vi "ST5 Read Param.vi"(6 "Facteur Dir":bool, 8 "error in (no error)":errorcluster, 9 "Facteur Pas":dbl=1500.0, 10 "Parameters":u16(ring) items=["All", "Velocity", "Acceleration", "Deceleration", "Max Acceleration", "Position", "Step/Rev", "Alarm Code", "Status"], 11 "Port COM":refnum<visa-resource-name>) -> (0 "error out":errorcluster, 1 "Status":T1, 2 "Position":dbl caption="Position (mm)" min=0.0 max=119304.64 step=0.018 format="%#.4g", 3 "Port COM Out":refnum<visa-resource-name>, 4 "Speed Par":T2 {"Accél Max" min=0.167 max=5461.167 step=0.167 format="%#.3g"; "Décél" min=0.167 max=5461.167 step=0.167 format="%#.3g"; "Accél" min=0.167 max=5461.167 step=0.167 format="%#.3g"; "Vitesse (Tour/s)" min=0.0042 max=133.3333 step=0.0042 format="%#.4g"}, 5 "Résolution Pas":dbl, 7 "Alarme":u32)   [LabVIEW 2010]
doc: "Ce Vi envoie les chaînes de commande au contrôlleur de moteur ST5-Q et vérifie si une réponse se trouve dans le buffer du port série"
uses:
  <userlib>/ST5/StatesConst.ctl
panel:
  out "ScanFailed":bool
  out "Réponse":string
  out "Commande":string
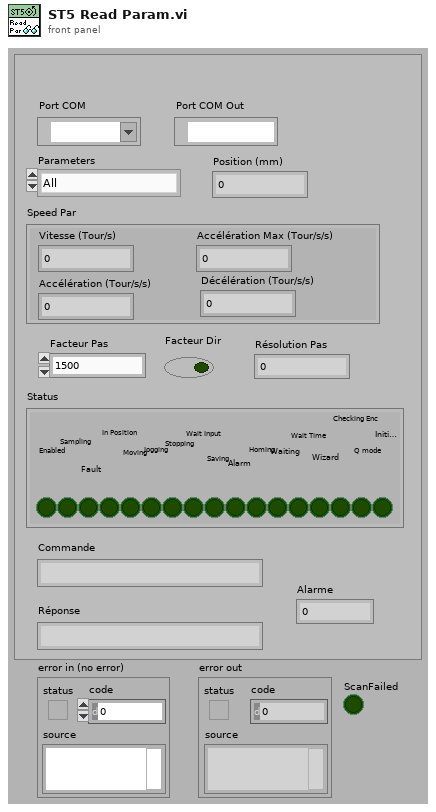
[diagram p1: front panel]
types:
  T1 = cluster{"Enabled":bool, "Sampling":bool, "Fault":bool, "In Position":bool, "Moving":bool, "Jogging":bool, "Stopping":bool, "Wait Input":bool, "Saving":bool, "Alarm":bool, "Homing":bool, "Waiting":bool, "Wait Time":bool, "Wizard":bool, "Checking Enc":bool, "Q mode":bool, "Initializing":bool}
  T2 = cluster{"Vitesse (Tour/s)":dbl, "Accél":dbl, "Décél":dbl, "Accél Max":dbl}
  T3 = typedef "StatesConst.ctl" = enum16{"SendCom", "Read", "End"}
  T4 = cluster{"Boolean array[0]":bool, "Boolean array[1]":bool, "Boolean array[2]":bool, "Boolean array[3]":bool, "Boolean array[4]":bool, "Boolean array[5]":bool, "Boolean array[6]":bool, "Boolean array[7]":bool, "Boolean array[8]":bool, "Boolean array[9]":bool, "Boolean array[10]":bool, "Boolean array[11]":bool, "Boolean array[12]":bool, "Boolean array[13]":bool, "Boolean array[14]":bool, "Boolean array[15]":bool, "Boolean array[16]":bool}
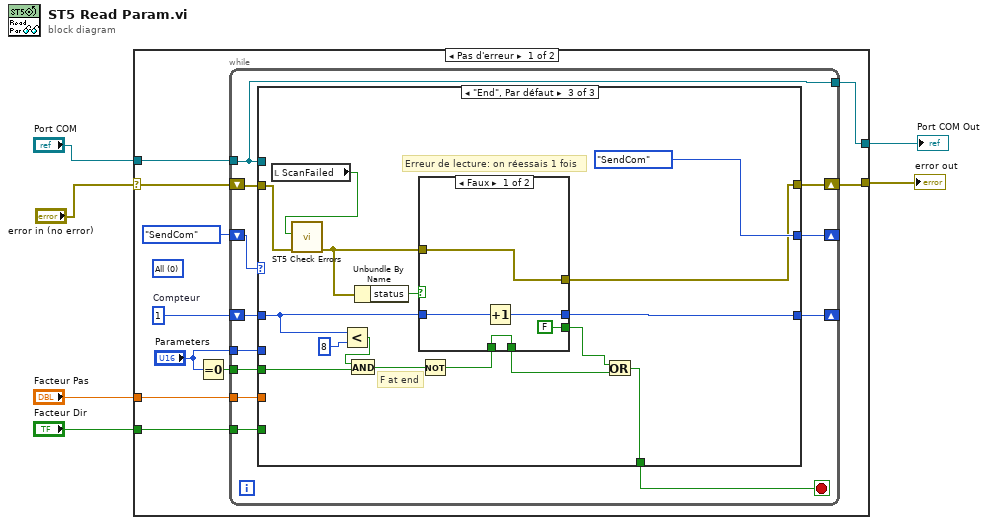
[diagram p0: block diagram]
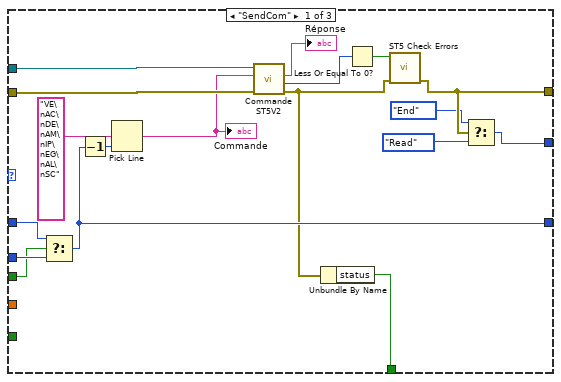
[diagram p2: hidden frame]
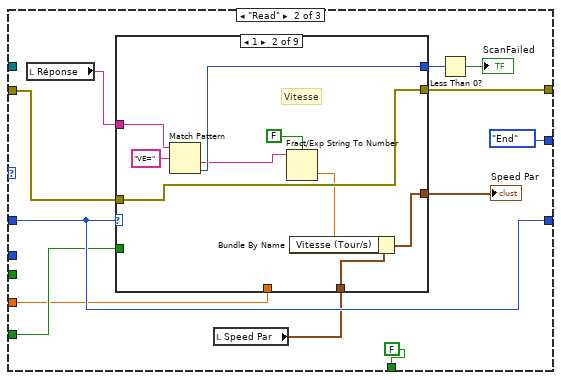
[diagram p3: hidden frame]
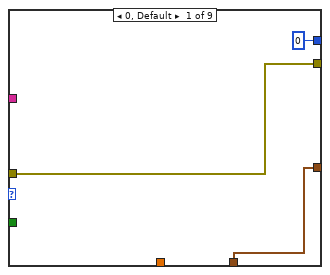
[diagram p4: hidden frame]
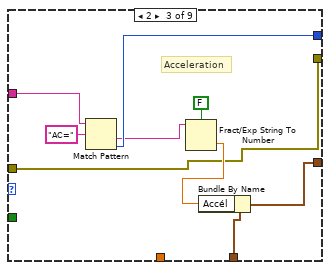
[diagram p5: hidden frame]
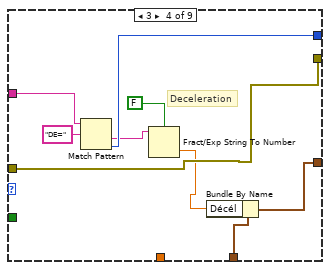
[diagram p6: hidden frame]
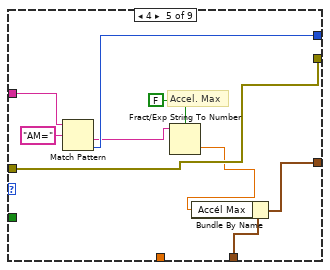
[diagram p7: hidden frame]
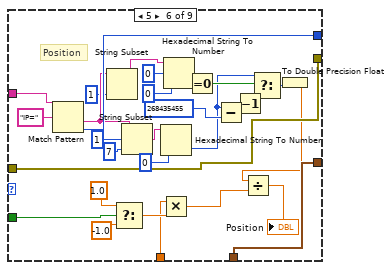
[diagram p8: hidden frame]
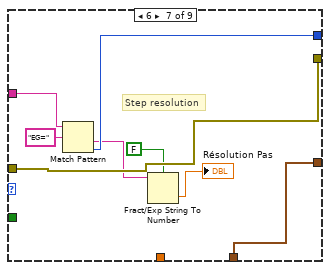
[diagram p9: hidden frame]
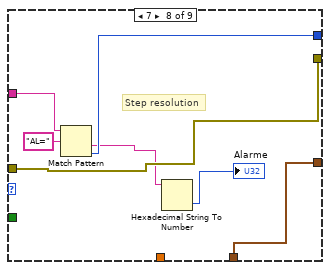
[diagram p10: hidden frame]
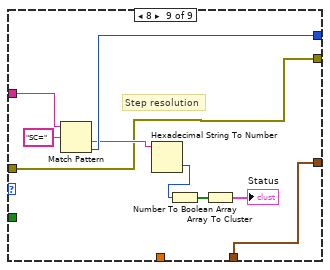
[diagram p11: hidden frame]
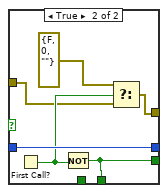
[diagram p12: hidden frame]
diagram:
  n1 = case shown="Pas d'erreur" "error in (no error)" {
    selector: "error in (no error)" -> [w15 w179]
    tunnel: "Port COM" -> [w16 w178]
    tunnel: [w7 w179] -> w4
    tunnel: [w10 w178] -> w3
    tunnel: "Facteur Dir" -> [w9 _]
    tunnel: "Facteur Pas" -> [w8 _]
    frame No Error {
      (unwired) u16 0 items=["All", "Velocity", "Acceleration", "Deceleration", "Max Acceleration", "Position"] ("Parameters")
      w14 = u16 1  # Compteur
      n2 = Equal To 0?(x="Parameters") -> (x = 0?=w11:bool)
      n3 = while {
        tunnel: w16 -> [w20]
        shift-right: [w17] -> w7
        shift-left: w15 -> [w28]
        shift-right: [w26] -> _
        shift-left: StatesConst."SendCom" ("Énum") -> [w27]
        tunnel: "Parameters" -> [w24]
        tunnel: w11 -> [w23]
        shift-right: [w22] -> _
        shift-left: w14 -> [w25]
        tunnel: [w20] -> w10
        tunnel: w9 -> [w19]
        tunnel: w8 -> [w18]
        stop <- w21 stop-if-true
        n4 = case shown="\"End\", Par défaut" w27 {
          tunnel: w20 -> [w39 _ _]
          tunnel: w28 -> [w38 w55 w155]
          tunnel: [w32 w54 w156] -> w17
          tunnel: [w29 StatesConst."End" ("Énum") StatesConst."SendCom" ("Énum")] -> w26
          tunnel: w25 -> [w43 w57 w162]
          tunnel: w24 -> [w45 _ _]
          tunnel: w23 -> [w44 _ w166]
          tunnel: [w41 w57 w163] -> w22
          tunnel: [w42 FALSE ("status") w158] -> w21
          tunnel: w19 -> [_ w52 _]
          tunnel: w18 -> [_ w51 _]
          frame "SendCom" {
            n5 = Select(t=w43, s=w44, f=w45) -> (s? t:f=w41:u16)
            n6 = Decrement(x=w41) -> (x-1=w40:u16)
            n7 = Pick Line(multi-line string="VE\nAC\nDE\nAM\nIP\nEG\nAL\nSC", line index=w40) -> (output string=w36:string)  [unwired: 1 in]
            "Commande" <- w36
            n8 = call <userlib>:"Commande ST5V2.vi"("error in (no error)"=w38, "Commande"=w36, "Port COM"=w39) -> ("error out"=w33:errorcluster, "Read"=w35:u32, "Réponse"=→"Réponse":string)  [unwired: 1 in, 1 out]
            n9 = Unbundle By Name(w33) -> ("status"=w42:bool)
            n10 = Less Or Equal To 0?(x=w35) -> (x <= 0?=w34:bool)
            n11 = call <userlib>:"ST5 Check Errors.vi"("error in (no error)"=w33, "Read=0"=w34) -> ("error out"=w32:errorcluster)  [unwired: 9 in]
            n12 = Select(t=StatesConst."End" ("Énum"), s=w32, f=StatesConst."Read" ("Énum")) -> (s? t:f=w29:T3)
          }
          frame "Read" {
            n13 = local read "Réponse"() -> (w56:string)
            n14 = local read "Speed Par"() -> (w50:T2)
            n15 = case shown="1" w57 {
              tunnel: w56 -> [_ w69 w79 w87 w96 w107 w132 w139 w148]
              tunnel: w55 -> [w60 w65 w72 w83 w91 w116 w130 w137 w142]
              tunnel: [w60 w65 w72 w83 w91 w116 w130 w137 w142] -> w54
              tunnel: w52 -> [_ _ _ _ _ w121 _ _ _]
              tunnel: w51 -> [_ _ _ _ _ w120 _ _ _]
              tunnel: w50 -> [w61 w68 w77 w86 w95 w118 w133 w140 w149]
              tunnel: [w61 w67 w76 w85 w94 w118 w133 w140 w149] -> w49
              tunnel: [0 ("offset past match") w66 w75 w84 w93 w117 w131 w138 w145] -> w48
              frame 0, Default {
              }
              frame 1 {
                # "Vitesse"
                n16 = Match Pattern(string=w69, regular expression="VE=") -> (after substring=w64:string, offset past match=w66:i32)  [unwired: 1 in, 2 out]
                n17 = Fract/Exp String To Number(use system decimal point (T)=FALSE ("utiliser le séparateur décimal du système (V)"), string=w64) -> (number=w63:dbl)  [unwired: 2 in, 1 out]
                n18 = Bundle By Name(cluster=w68, "Vitesse (Tour/s)"=w63) -> (w67:T2)
              }
              frame 2 {
                # "Acceleration"
                n19 = Match Pattern(string=w79, regular expression="AC=") -> (after substring=w74:string, offset past match=w75:i32)  [unwired: 1 in, 2 out]
                n20 = Fract/Exp String To Number(use system decimal point (T)=FALSE ("utiliser le séparateur décimal du système (V)"), string=w74) -> (number=w73:dbl)  [unwired: 2 in, 1 out]
                n21 = Bundle By Name(cluster=w77, "Accél"=w73) -> (w76:T2)
              }
              frame 3 {
                # "Deceleration"
                n22 = Match Pattern(string=w87, regular expression="DE=") -> (after substring=w82:string, offset past match=w84:i32)  [unwired: 1 in, 2 out]
                n23 = Fract/Exp String To Number(use system decimal point (T)=FALSE ("utiliser le séparateur décimal du système (V)"), string=w82) -> (number=w81:dbl)  [unwired: 2 in, 1 out]
                n24 = Bundle By Name(cluster=w86, "Décél"=w81) -> (w85:T2)
              }
              frame 4 {
                # "Accel. Max"
                n25 = Match Pattern(string=w96, regular expression="AM=") -> (after substring=w92:string, offset past match=w93:i32)  [unwired: 1 in, 2 out]
                n26 = Fract/Exp String To Number(use system decimal point (T)=FALSE ("utiliser le séparateur décimal du système (V)"), string=w92) -> (number=w90:dbl)  [unwired: 2 in, 1 out]
                n27 = Bundle By Name(cluster=w95, "Accél Max"=w90) -> (w94:T2)
              }
              frame 5 {
                # "Position"
                n28 = Match Pattern(string=w107, regular expression="IP=") -> (after substring=w100:string, offset past match=w117:i32)  [unwired: 1 in, 2 out]
                n29 = String Subset(string=w100, length (rest)=1 ("longueur (reste)")) -> (substring=w98:string)  [unwired: 1 in]
                n30 = Select(t=1.0 ("pas/mm"), s=w121, f=-1.0 ("pas/mm")) -> (s? t:f=w122:dbl)
                n31 = String Subset(string=w100, offset (0)=1, length (rest)=7 ("longueur (reste)")) -> (substring=w112:string)
                n32 = Hexadecimal String To Number(string=w112, default (0uL)=0 ("valeur par défaut (0 U32)")) -> (number=w103:i32)  [unwired: 1 in, 1 out]
                n33 = Multiply(x=w120, y=w122) -> (x*y=w119:dbl)
                n34 = Hexadecimal String To Number(string=w98, offset=0, default (0uL)=0 ("valeur par défaut (0 U32)")) -> (number=w114:i32)  [unwired: 1 out]
                n35 = Equal To 0?(x=w114) -> (x = 0?=w113:bool)
                n36 = Subtract(x=w103, y=268435455) -> (x-y=w105:i32)
                n37 = Decrement(x=w105) -> (x-1=w101:i32)
                n38 = Select(t=w103, s=w113, f=w101) -> (s? t:f=w110:i32)
                n39 = To Double Precision Float(number=w110) -> (double precision float=w109:dbl)
                n40 = Divide(x=w109, y=w119) -> (x/y=→"Position":dbl)
              }
              frame 6 {
                # "Step resolution"
                n41 = Match Pattern(string=w132, regular expression="EG=") -> (after substring=w129:string, offset past match=w131:i32)  [unwired: 1 in, 2 out]
                n42 = Fract/Exp String To Number(use system decimal point (T)=FALSE ("utiliser le séparateur décimal du système (V)"), string=w129) -> (number=→"Résolution Pas":dbl)  [unwired: 2 in, 1 out]
              }
              frame 7 {
                # "Step resolution"
                n43 = Match Pattern(string=w139, regular expression="AL=") -> (after substring=w136:string, offset past match=w138:i32)  [unwired: 1 in, 2 out]
                n44 = Hexadecimal String To Number(string=w136) -> (number=→"Alarme":u32)  [unwired: 2 in, 1 out]
              }
              frame 8 {
                # "Step resolution"
                n45 = Match Pattern(string=w148, regular expression="SC=") -> (after substring=w144:string, offset past match=w145:i32)  [unwired: 1 in, 2 out]
                n46 = Hexadecimal String To Number(string=w144) -> (number=w143:u32)  [unwired: 2 in, 1 out]
                n47 = Number To Boolean Array(number=w143) -> (Boolean array=w146:bool[])
                n48 = Array To Cluster(array=w146) -> (cluster=→"Status":T4)
              }
            }
            "Speed Par" <- w49
            n49 = Less Than 0?(x=w48) -> (x < 0?=→"ScanFailed":bool)
          }
          frame "End", Default {
            # "F at end"
            # "Erreur de lecture: on réessais 1 fois"
            n50 = local read "ScanFailed"() -> (w153:bool)
            n51 = call <userlib>:"ST5 Check Errors.vi"("error in (no error)"=w155, "Scan failed"=w153) -> ("error out"=w154:errorcluster)  [unwired: 9 in]
            n52 = Less?(x=w162, y=u16 8) -> (x < y?=w165:bool)
            n53 = And(x=w165, y=w166) -> (x .and. y?=w161:bool)
            n54 = Unbundle By Name(w154) -> ("status"=w159:bool)
            n55 = Not(x=w161) -> (.not. x?=w152:bool)
            n56 = case shown="Faux" w159 {
              tunnel: [w171 w177] -> w163
              tunnel: w162 -> [w170 w177]
              tunnel: [FALSE w172] -> w157
              tunnel: w154 -> [w169 w175]
              tunnel: [w169 w174] -> w156
              tunnel: w152 -> [w168 _]
              tunnel: [w168 w172] -> w151
              frame False {
                n57 = Increment(x=w170) -> (x+1=w171:u16)
              }
              frame True {
                n58 = First Call?() -> (First Call?: T/F=w176:bool)
                n59 = Not(x=w176) -> (.not. x?=w172:bool)
                n60 = Select(t=errorcluster {"status"=FALSE, "code"=0, "source"=""} ("error IO"), s=w176, f=w175) -> (s? t:f=w174:errorcluster)
              }
            }
            n61 = Or(x=w157, y=w151) -> (x .or. y?=w158:bool)
          }
        }
      }
    }
    frame Error {
    }
  }
  "error out" <- w4
  "Port COM Out" <- w3
